vi "Binary2ASCII.vi"() -> ()   [LabVIEW 2014]
uses:
  <userlib>/Nanonis Prog Interface V5/Nanonis Prog Interface.lvlib
  <userlib>/Nanonis Prog Interface V5/File/Binary_SpectroscopyFile-Config.ctl
panel:
  out "Config":T1
  out "Global Attributes":string[][](table)
  out "data":sgl[][](array[numeric]) format="%#_4p"
  out "error out Write file":errorcluster
  out "error out Read file":errorcluster
  in  "Binary Spectroscopy File":path
  # "This VI takes a 3ds file as input to create a new 3ds file with the derived signals.\nIf the source files contains I/V curves this VI will create a new file containing calculated dI/dV curves.\nThe derivative is calculated by determining the slope of a piece-wise linear fit to the input signals. Due to the nature of this derivative some points at the beginning and at the end will be cut, so the resulting curves will have less points and the sweep signal limits will be different."
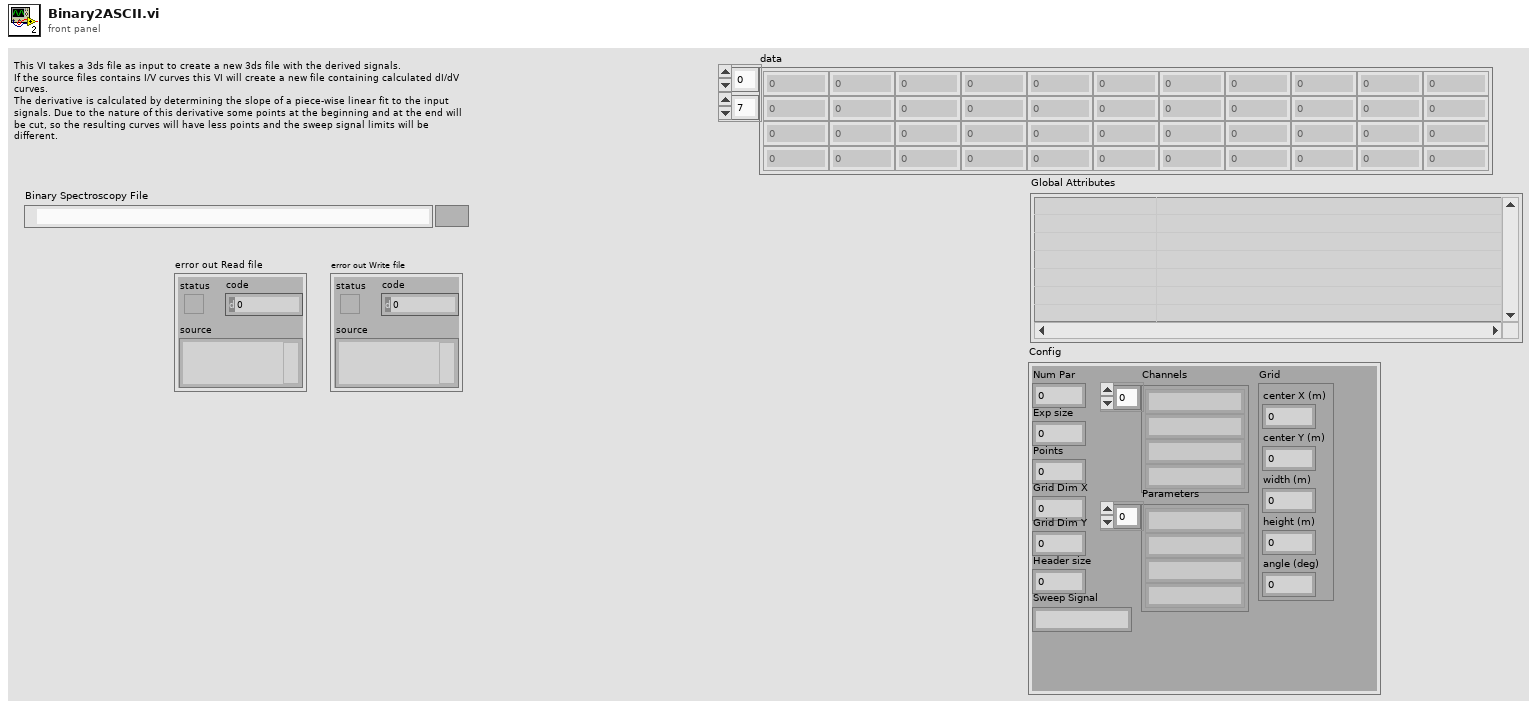
[diagram p1: front panel]
types:
  T1 = typedef "Nanonis Prog Interface.lvlib/Binary_SpectroscopyFile-Config.ctl" = cluster{"Num Par":i32, "Exp size":i32, "Points":i32, "Grid Dim X":i32, "Grid Dim Y":i32, "Header size":i32, "Channels":string[], "Parameters":string[], "Sweep Signal":string, "Grid":cluster{"center X (m)":sgl, "center Y (m)":sgl, "width (m)":sgl, "height (m)":sgl, "angle (deg)":sgl}}
  T2 = cluster{"center X (m)":sgl, "center Y (m)":sgl, "width (m)":sgl, "height (m)":sgl, "angle (deg)":sgl}
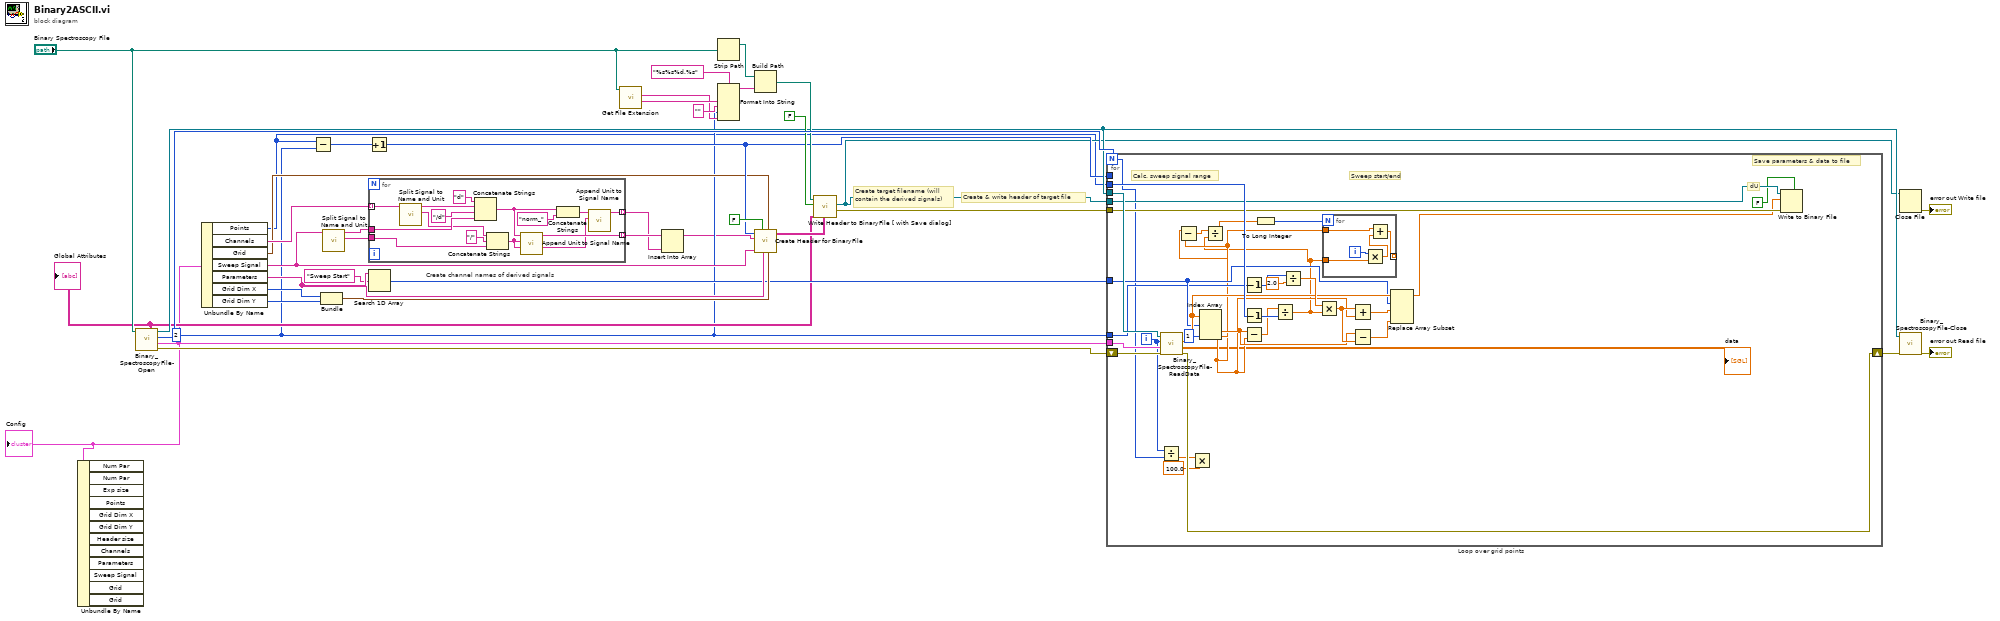
[diagram p0: block diagram]
diagram:
  w7 = u16 2 ("Fit length for derivative")
  # "Create & write header of target file"
  # "Create target filename (will contain the derived signals)"
  n1 = call <userlib>:"Binary_SpectroscopyFile-Open.vi"("Binary Spectroscopy File"="Binary Spectroscopy File") -> ("error out"=w39:errorcluster, "Config"=w2:T1, "Number of Experiments"=w40:i32, "File ref"=w28:refnum<file>, "Global Attributes"=w13:string[][])  [unwired: 6 in]
  "Global Attributes" <- w13
  "Config" <- w2
  n2 = Unbundle By Name(w2) -> ("Parameters"=w1:string[])  [unwired: 11 out]
  n3 = Unbundle By Name(w2) -> ("Points"=w3:i32, "Channels"=w27:string[], "Grid"=w18:T2, "Sweep Signal"=w26:string, "Parameters"=w22:string[], "Grid Dim X"=w37:i32, "Grid Dim Y"=w36:i32)
  n4 = Subtract(x=w3, y=w7) -> (x-y=w23:i32)
  n5 = Bundle("Grid Dim X"=w37, "Grid Dim Y"=w36) -> (w35:cluster{"Grid Dim X":i32, "Grid Dim Y":i32})  [unwired: 1 in]
  n6 = call <userlib>:"Split Signal to Name and Unit.vi"("Name with unit"=w26) -> ("Unit"=w24:string, "Name"=w25:string)  [unwired: 5 in]
  n7 = Increment(x=w23) -> (x+1=w19:i32)
  n8 = for "Create channel names of derived signals" {
    tunnel: w27 -> [w54] mode=indexing
    tunnel: w25 -> [w50]
    tunnel: w24 -> [w47]
    tunnel: [w46] -> w5 mode=indexing
    tunnel: [w41] -> w4 mode=indexing
    n9 = call <userlib>:"Split Signal to Name and Unit.vi"("Name with unit"=w54) -> ("Unit"=w49:string, "Name"=w53:string)  [unwired: 5 in]
    n10 = Concatenate Strings("d" ("string"), w53, "/d" ("string"), w50) -> (w44:string)
    n11 = Concatenate Strings(w49, "/" ("string"), w47) -> (w45:string)
    n12 = call <userlib>:"Append Unit to Signal Name.vi"("Unit"=w45, "Name"=w44) -> ("Name with unit"=w46:string)  [unwired: 5 in]
    n13 = Concatenate Strings(w44, "norm_" ("string")) -> (w43:string)
    n14 = call <userlib>:"Append Unit to Signal Name.vi"("Unit"=w45, "Name"=w43) -> ("Name with unit"=w41:string)  [unwired: 5 in]
  }
  n15 = Search 1D Array(1D array=w22, element="Sweep Start") -> (index of element=w20:i32)  [unwired: 1 in]
  n16 = call <vilib>:"Get File Extension.vi"("file"="Binary Spectroscopy File") -> ("filename without extension"=w10:string, "lowercase file extension"=w9:string)  [unwired: 7 in, 2 out]
  n17 = Insert Into Array(array=w5, new element=w4) -> (w6:string[])  [unwired: 1 in]
  n18 = Strip Path(path="Binary Spectroscopy File") -> (stripped path=w33:path)  [unwired: 1 out]
  n19 = Format Into String(format string="%s%s%d.%s", w10, "" ("string"), w7, w9) -> (resulting string=w8:string)  [unwired: 2 in, 1 out]
  n20 = Build Path(base path=w33, name or relative path=w8) -> (appended path=w32:path)
  n21 = call <userlib>:"Create Header for BinaryFile.vi"("Grid points"=w35, "Grid param"=w18, "Fixed parameters"=w22, "Backward sweep"=FALSE, "Sweep signal"=w26, "Channels"=w6, "Points per sweep"=w19) -> ("Header (fixed attributes)"=w30:string[][])  [unwired: 4 in]
  n22 = call <userlib>:"Write Header to BinaryFile [ with Save dialog].vi"("Fixed Attributes"=w30, "Attributes in"=w13, "Show Dialog? (T)"=FALSE, "Filename"=w32) -> ("Error out"=w17:errorcluster, "File ref"=w16:refnum<file>)  [unwired: 4 in, 2 out]
  n23 = for "Loop over grid points" {
    N: w40 -> [w57]
    tunnel: w28 -> [w87]
    tunnel: w2 -> [w86]
    shift-right: [w84] -> w29
    shift-left: w39 -> [w85]
    tunnel: w16 -> [w72]
    tunnel: w7 -> [w69]
    tunnel: w20 -> [w75]
    tunnel: w3 -> [w83]
    tunnel: w19 -> [_]
    tunnel: w17 -> [w71]
    i -> [w58]
    # "dU"
    # "Sweep start/end"
    # "Save parameters & data to file"
    # "Calc. sweep signal range"
    n24 = call <userlib>:"Binary_SpectroscopyFile-ReadData.vi"("error in"=w85, "Config"=w86, "Experiment to read (Index)"=w58, "File ref In"=w87) -> ("error out"=w84:errorcluster, "data"=→"data":sgl[][], "Parameter values"=w76:sgl[])  [unwired: 4 in, 1 out]
    n25 = Divide(x=w58, y=w57) -> (x/y=w59:dbl)
    n26 = Multiply(x=w59, y=100.0) -> ()  [unwired: 1 out]
    n27 = Index Array(array=w76, index #1=w75, index #3=1 ("index")) -> (element #1=w64:sgl, element #2=w67:sgl, element #3=w65:sgl)  [unwired: 1 in]
    n28 = Subtract(x=w65, y=w64) -> (x-y=w63:sgl)
    n29 = Decrement(x=w69) -> (x-1=w80:u16)
    n30 = Decrement(x=w83) -> (x-1=w82:i32)
    n31 = Subtract(x=w67, y=w64) -> (x-y=w81:sgl)
    n32 = Divide(x=w81, y=w82) -> (x/y=w62:sgl)
    n33 = Divide(x=w63, y=w62) -> (x/y=w61:sgl)
    n34 = To Long Integer(number=w61) -> (32bit integer=w60:i32)
    n35 = Divide(x=w80, y=sgl 2.0) -> (x/y=w78:sgl)
    n36 = Multiply(x=w78, y=w62) -> (x*y=w77:sgl)
    n37 = for {
      N: w60 -> [_]
      tunnel: w62 -> [w91]
      tunnel: [w89] -> _ mode=indexing
      tunnel: w64 -> [w88]
      i -> [w92]
      n38 = Multiply(x=w92, y=w91) -> (x*y=w90:sgl)
      n39 = Add(x=w88, y=w90) -> (x+y=w89:sgl)
    }
    n40 = Add(x=w77, y=w64) -> (x+y=w74:sgl)
    n41 = Subtract(x=w67, y=w77) -> (x-y=w73:sgl)
    n42 = Replace Array Subset(array=w76, new element #1=w74, index #1=w75, new element #2=w73) -> (w68:sgl[])  [unwired: 1 in]
    n43 = Write to Binary File(file (use dialog)=w72, data=w68, error in=w71, 5:FALSE ("prepend array or string size? (T)")) -> ()  [unwired: 2 in, 3 out]
  }
  n44 = Close File(refnum=w16) -> (error out=→"error out Write file":errorcluster)  [unwired: 1 in, 1 out]
  n45 = call <userlib>:"Binary_SpectroscopyFile-Close.vi"("error in"=w29, "File ref"=w28) -> ("error out"=→"error out Read file":errorcluster)  [unwired: 9 in]
